vi "Begin.vi"(8 "error in":errorcluster) -> (0 "error out":errorcluster)   [LabVIEW 2017]
doc: "Called before other user functions, this VI is expected to open initial I/O refnums, load in file data, and do all program initialization. Notice that the <B>error out</B> terminal is simply used for data flow. Wiring it to other structures or subVIs ensures that this VI runs first."
uses:
  <vilib>/Rock Robotics/WPI/DriverStation/WPI_DriverStationRobotMode2.ctl
  <vilib>/Rock Robotics/WPI/Joystick/WPI_JoystickDeviceEnum.ctl
  <vilib>/Rock Robotics/WPI/ThirdParty/Phoenix-LabVIEW/Motor Controller/Controls/CTRE_Phoenix_MotorControl_ControlMode.ctl
  <vilib>/Rock Robotics/WPI/ThirdParty/Phoenix-LabVIEW/Motor Controller/Controls/CTRE_Phoenix_MotorControl_NeutralMode.ctl
  <vilib>/Rock Robotics/WPI/ThirdParty/Phoenix-LabVIEW/Motor Controller/Controls/CTRE_Phoenix_MotorControl_FeedbackDevice.ctl
  <vilib>/Rock Robotics/SystemInterfaces/spilib/spi_bus.ctl
  <vilib>/Rock Robotics/WPI/Solenoid/WPI_SolenoidChannel.ctl
  <vilib>/Rock Robotics/SystemInterfaces/DIO/FPGA_DIOChannel.ctl
  Robot Global Data.vi
  <vilib>/Rock Robotics/Network Tables/NT Write Numeric Array.vi
  <vilib>/Rock Robotics/WPI/Utilities/WPI_GetSetVariantRefNum.vi
  <vilib>/Rock Robotics/WPI/Gyro/WPI_GyroXRS450_SPI_Open.vi
  <vilib>/Rock Robotics/WPI/Switch/WPI_SwitchOpenLimit.vi
  <vilib>/Rock Robotics/WPI/Solenoid/WPI_SolenoidOpenDouble.vi
  <vilib>/Rock Robotics/Network Tables/NT Write String Array.vi
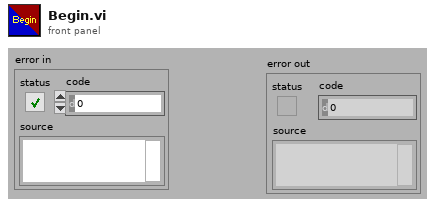
[diagram p1: front panel]
types:
  T1 = typedef "WPI_SolenoidChannel.ctl" = enum8{"Solenoid 0", "Solenoid 1", "Solenoid 2", "Solenoid 3", "Solenoid 4", "Solenoid 5", "Solenoid 6", "Solenoid 7", "Invalid"}
  T2 = typedef "FPGA_DIOChannel.ctl" = enum8{"DIO 0", "DIO 1", "DIO 2", "DIO 3", "DIO 4", "DIO 5", "DIO 6", "DIO 7", "DIO 8", "DIO 9", "DIO MXP 0", "DIO MXP 1", "DIO MXP 2", "DIO MXP 3", "DIO MXP 4", "DIO MXP 5", "DIO MXP 6", "DIO MXP 7", "DIO MXP 8", "DIO MXP 9", "DIO MXP 10", "DIO MXP 11", "DIO MXP 12", "DIO MXP 13", "DIO MXP 14", "DIO MXP 15", "SPI Port CS1", "SPI Port CS2", "SPI Port CS3", "SPI Port MISO", "SPI Port MOSI", "Invalid"}
  T3 = typedef "spi_bus.ctl" = enum16{"SPI On-Board, CS0", "SPI On-Board, CS1", "SPI On-Board, CS2", "SPI On-Board, CS3", "SPI MXP", "Invalid"}
  T4 = typedef "CTRE_Phoenix_MotorControl_FeedbackDevice.ctl" = i8
  T5 = typedef "CTRE_Phoenix_MotorControl_NeutralMode.ctl" = enum8{"EEPROMSetting", "Override to Coast", "Override to Brake"}
  T6 = typedef "CTRE_Phoenix_MotorControl_ControlMode.ctl" = u16
  T7 = typedef "WPI_JoystickDeviceEnum.ctl" = enum16{"USB 0", "USB 1", "USB 2", "USB 3", "USB 4", "USB 5"}
  T8 = typedef "WPI_DriverStationRobotMode2.ctl" = enum16{"Autonomous Disabled", "Autonomous Enabled", "Teleop Disabled", "Teleop Enabled", "Disconnected", "Finish", "Test Disabled", "Test Enabled", "Emergency Stopped"}
  T9 = typedef "WPI_SolenoidDevRef.ctl" = cluster{"DevStatus":errorcluster, "Pneumatics Control Module":u8, "Forward Solenoid Channel":T1, "Reverse Solenoid Channel":T1}
  T10 = typedef "WPI_JoystickDevRef.ctl" = cluster{"Device":T7}
  T11 = typedef "WPI_SwitchDevRef.ctl" = cluster{"DevStatus":errorcluster, "DIO Channel":T2, "CntIndex":T12, "Normally Closed":bool}
  T12 = typedef "FPGA_CounterCtrSystemIndex.ctl" = enum8{"Ctr 0", "Ctr 1", "Ctr 2", "Ctr 3", "Ctr 4", "Ctr 5", "Ctr 6", "Ctr 7", "Invalid"}
  T13 = typedef "WPI_MotorControlDeviceRef.ctl" = cluster{"DeviceStatus":errorcluster, "Type":T14, "PWM":cluster{"PWM Channel":T15, "DeadBand":T16}, "CAN":cluster{"Device Number":u8, "SetOutput VI Ref":variant, "GetOutput VI Ref":variant, "Enable VI Ref":variant, "Disable VI Ref":variant, "Data":variant}, "Invert":bool, "DIO PWM":cluster{"PWM \"Enable\" Channel":T15, "DIOChannel":T2, "PWM Rate":dbl}}
  T14 = typedef "WPI_MotorControlType.ctl" = enum16{"PWM", "CAN", "DIO PWM"}
  T15 = typedef "FPGA_DIOPWMChannel.ctl" = enum8{"PWM 0", "PWM 1", "PWM 2", "PWM 3", "PWM 4", "PWM 5", "PWM 6", "PWM 7", "PWM 8", "PWM 9", "PWM MXP 0", "PWM MXP 1", "PWM MXP 2", "PWM MXP 3", "PWM MXP 4", "PWM MXP 5", "PWM MXP 6", "PWM MXP 7", "PWM MXP 8", "PWM MXP 9", "Invalid"}
  T16 = typedef "WPI_PWMDeadband.ctl" = cluster{"Name":string, "maxPositivePwm":i32, "minPositivePwm":i32, "centerPwm":i32, "maxNegativePwm":i32, "minNegativePwm":i32, "angularRange":u16}
  T17 = typedef "WPI_GyroDevRef.ctl" = cluster{"DevStatus":errorcluster, "Analog Channel":T18, "Gain (VoltsPerDegree/Second)":dbl, "Gyro Type":enum16{"Analog", "XRS450"}, "Handle":i32, "SPI Bus":T3, "Device Found":bool, "Sample Rate":dbl, "Calibrate On Open":bool, "Offset":dbl}
  T18 = typedef "FPGA_AIChannel.ctl" = enum8{"AI 0", "AI 1", "AI 2", "AI 3", "AI MXP 0", "AI MXP 1", "AI MXP 2", "AI MXP 3", "Invalid"}
  T19 = typedef "WPI_CompressorDevRef.ctl" = cluster{"DevStatus":errorcluster, "Pneumatics Control Module":u8}
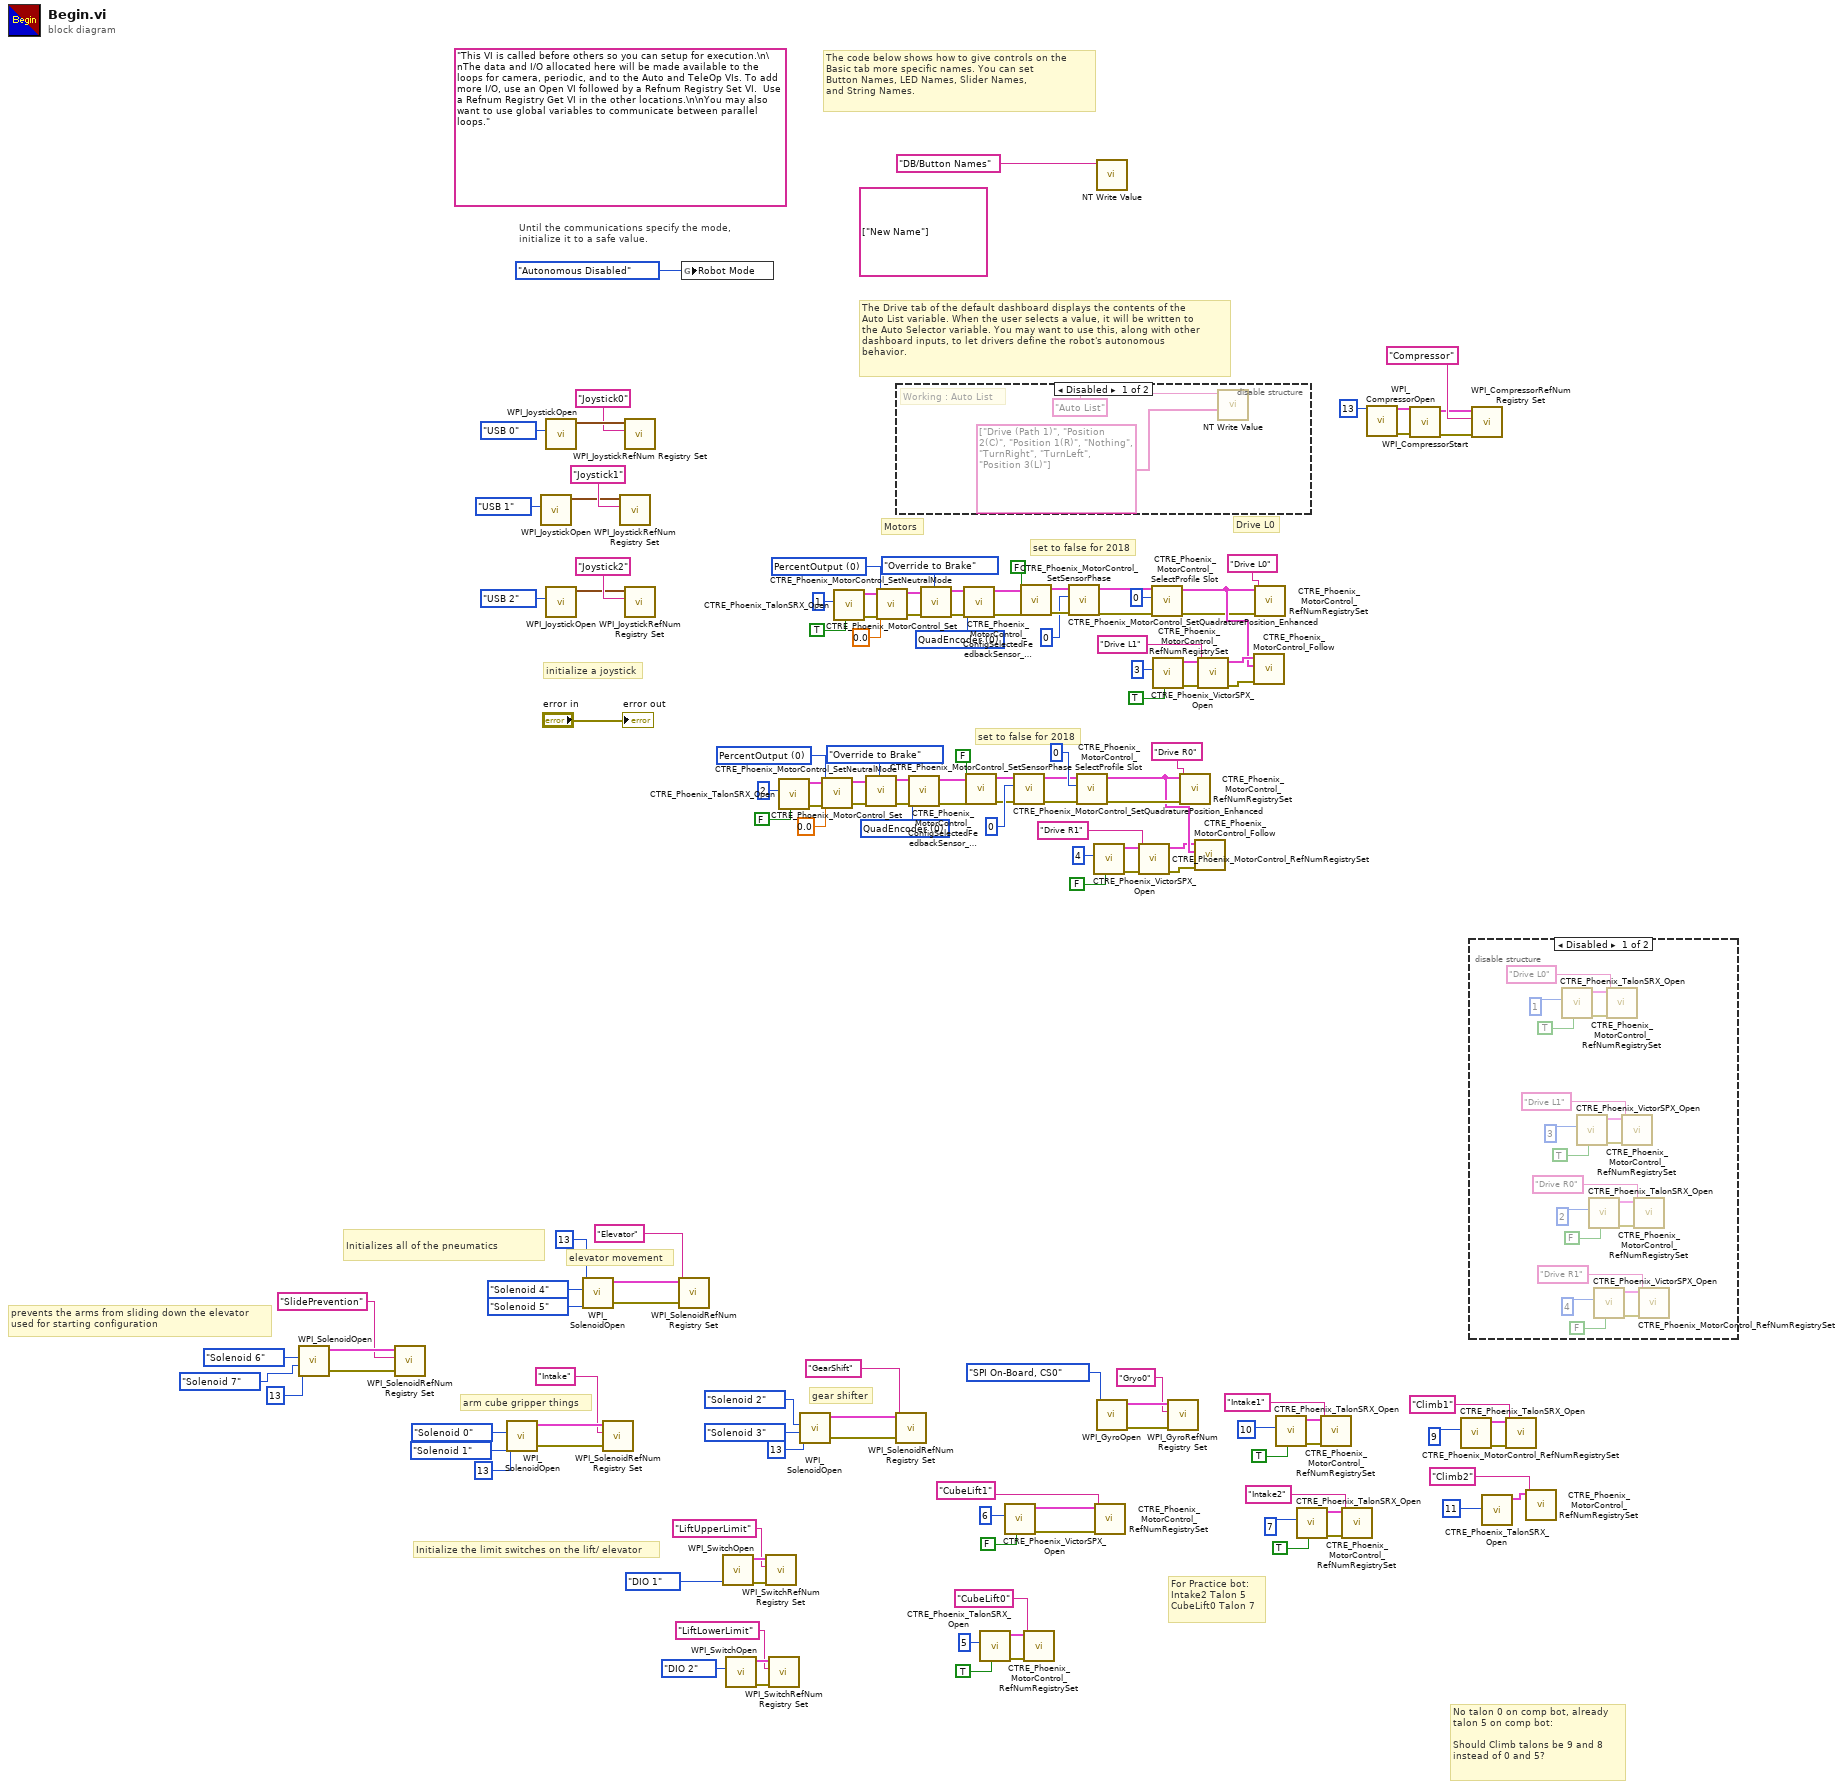
[diagram p0: block diagram]
diagram:
  w93 = T4 0 items=["None"=-1, "QuadEncoder"=0, "Analog"=2, "Tachometer"=4, "Pulse Width Encoded Position"=8, "Sensor Sum (S0 + S1)"=9, "Sensor Difference (D0 - D1)"=10, "Remote Source 0"=11, "Remote Source 1"=12, "Software Emulated"=15] ("Feedback Device")
  w88 = T6 0 items=["PercentOutput"=0, "Position"=1, "Velocity"=2, "Current"=3, "Follower"=5, "MotionProfile"=6, "MotionMagic"=7, "MotionMagicArc"=8, "MotionProfileArc"=10, "Disabled"=15] ("Control Mode")
  w112 = T4 0 items=["None"=-1, "QuadEncoder"=0, "Analog"=2, "Tachometer"=4, "Pulse Width Encoded Position"=8, "Sensor Sum (S0 + S1)"=9, "Sensor Difference (D0 - D1)"=10, "Remote Source 0"=11, "Remote Source 1"=12, "Software Emulated"=15] ("Feedback Device")
  w117 = T6 0 items=["PercentOutput"=0, "Position"=1, "Velocity"=2, "Current"=3, "Follower"=5, "MotionProfile"=6, "MotionMagic"=7, "MotionMagicArc"=8, "MotionProfileArc"=10, "Disabled"=15] ("Control Mode")
  (unwired) string[] ["New Name"]
  (unwired) "This VI is called before others so you can setup for execution.\n\nThe data and I/O allocated here will be made available to the loops for camera, periodic, and to the Auto and TeleOp VIs. To add more I/O, use an Open VI followed by a Refnum Registry Set VI.  Use a Refnum Registry Get VI in the other locations.\n\nYou may also want to use global variables to communicate between parallel loops."
  # "prevents the arms from sliding down the elevator\nused for starting configuration"
  # "No talon 0 on comp bot, already\ntalon 5 on comp bot:\n\nShould Climb talons be 9 and 8\ninstead of 0 and 5?"
  # "gear shifter"
  # "arm cube gripper things"
  # "elevator movement"
  # "Initialize the limit switches on the lift/ elevator"
  # "Initializes all of the pneumatics"
  # "For Practice bot:\nIntake2 Talon 5\nCubeLift0 Talon 7"
  # "set to false for 2018"
  # "set to false for 2018"
  # "Drive L0"
  # "Motors"
  # "The Drive tab of the default dashboard displays the contents of the\nAuto List variable. When the user selects a value, it will be written to\nthe Auto Selector variable. You may want to use this, along with other\ndashboard inputs, to let drivers define the robot's autonomous\nbehavior."
  # "The code below shows how to give controls on the\nBasic tab more specific names. You can set\nButton Names, LED Names, Slider Names,\nand String Names."
  # "initialize a joystick"
  # "Until the communications specify the mode,\ninitialize it to a safe value."
  n1 = call-poly <vilib>:"WPI_SolenoidOpen.vi"("Reverse Solenoid Channel"=WPI_SolenoidChannel."Solenoid 7" ("Forward Solenoid Channel"), "Forward Solenoid Channel"=WPI_SolenoidChannel."Solenoid 6", "Pneumatics Control Module (0)"=u8 13) -> ("error out"=w5:errorcluster, "SolenoidDevRef"=w7:T9)  [unwired: 7 in]
  n2 = call <vilib>:"WPI_SolenoidRefNum Registry Set.vi"("error in (no error)"=w5, "refnum name"="SlidePrevention", "SolenoidDevRef"=w7) -> ()  [unwired: 7 in, 2 out]
  n3 = call-poly <vilib>:"WPI_SolenoidOpen.vi"("Reverse Solenoid Channel"=WPI_SolenoidChannel."Solenoid 1", "Forward Solenoid Channel"=WPI_SolenoidChannel."Solenoid 0", "Pneumatics Control Module (0)"=u8 13) -> ("error out"=w8:errorcluster, "SolenoidDevRef"=w30:T9)  [unwired: 7 in]
  n4 = call <vilib>:"WPI_JoystickOpen.vi"("JoystickDevice"=WPI_JoystickDeviceEnum."USB 1") -> ("JoystickDevRef"=w141:T10)  [unwired: 10 in]
  n5 = call <vilib>:"WPI_JoystickOpen.vi"("JoystickDevice"=WPI_JoystickDeviceEnum."USB 0") -> ("JoystickDevRef"=w136:T10)  [unwired: 10 in]
  n6 = call <vilib>:"WPI_JoystickOpen.vi"("JoystickDevice"=WPI_JoystickDeviceEnum."USB 2") -> ("JoystickDevRef"=w133:T10)  [unwired: 10 in]
  n7 = call-poly <vilib>:"WPI_SolenoidOpen.vi"("Reverse Solenoid Channel"=WPI_SolenoidChannel."Solenoid 5", "Forward Solenoid Channel"=WPI_SolenoidChannel."Solenoid 4", "Pneumatics Control Module (0)"=u8 13) -> ("error out"=w38:errorcluster, "SolenoidDevRef"=w37:T9)  [unwired: 7 in]
  n8 = call <vilib>:"WPI_SolenoidRefNum Registry Set.vi"("error in (no error)"=w8, "refnum name"="Intake", "SolenoidDevRef"=w30) -> ()  [unwired: 7 in, 2 out]
  n9 = call <vilib>:"WPI_JoystickRefNum Registry Set.vi"("refnum name"="Joystick1", "JoystickDevRef"=w141) -> ()  [unwired: 8 in, 2 out]
  n10 = call <vilib>:"WPI_JoystickRefNum Registry Set.vi"("refnum name"="Joystick0", "JoystickDevRef"=w136) -> ()  [unwired: 8 in, 2 out]
  n11 = call <vilib>:"WPI_JoystickRefNum Registry Set.vi"("refnum name"="Joystick2", "JoystickDevRef"=w133) -> ()  [unwired: 8 in, 2 out]
  n12 = call <vilib>:"WPI_SolenoidRefNum Registry Set.vi"("error in (no error)"=w38, "refnum name"="Elevator", "SolenoidDevRef"=w37) -> ()  [unwired: 7 in, 2 out]
  n13 = global write "Robot Global Data.vi" "Robot Mode"(WPI_DriverStationRobotMode2."Autonomous Disabled" ("Robot Mode")) -> ()
  n14 = call-poly <vilib>:"WPI_SwitchOpen.vi"("DIO Channel"=FPGA_DIOChannel."DIO 1") -> ("error out"=w27:errorcluster, "SwitchDevRef"=w26:T11)  [unwired: 9 in]
  n15 = call-poly <vilib>:"WPI_SwitchOpen.vi"("DIO Channel"=FPGA_DIOChannel."DIO 2") -> ("error out"=w24:errorcluster, "SwitchDevRef"=w23:T11)  [unwired: 9 in]
  n16 = call <vilib>:"WPI_SwitchRefNum Registry Set.vi"("error in (no error)"=w27, "refnum name"="LiftUpperLimit", "SwitchDevRef"=w26) -> ()  [unwired: 7 in, 2 out]
  n17 = call <vilib>:"WPI_SwitchRefNum Registry Set.vi"("error in (no error)"=w24, "refnum name"="LiftLowerLimit", "SwitchDevRef"=w23) -> ()  [unwired: 7 in, 2 out]
  n18 = call "CTRE_Phoenix_TalonSRX_Open.vi"("Invert"=FALSE, "Device Number"=u8 2) -> ("error out"=w85:errorcluster, "CAN Talon SRX Ref"=w84:T13)  [unwired: 8 in]
  n19 = call-poly <vilib>:"WPI_SolenoidOpen.vi"("Reverse Solenoid Channel"=WPI_SolenoidChannel."Solenoid 3", "Forward Solenoid Channel"=WPI_SolenoidChannel."Solenoid 2", "Pneumatics Control Module (0)"=u8 13) -> ("error out"=w31:errorcluster, "SolenoidDevRef"=w32:T9)  [unwired: 7 in]
  n20 = call <vilib>:"CTRE_Phoenix_MotorControl_Set.vi"("error in (no error)"=w85, "Output"=0.0, "Control Mode"=w88, "PhoenixMotorControlDevRef"=w84) -> ("error out"=w87:errorcluster, "PhoenixMotorControlDevRef"=w86:T13)  [unwired: 6 in]
  n21 = call "CTRE_Phoenix_TalonSRX_Open.vi"("Invert"=TRUE, "Device Number"=u8 1) -> ("error out"=w120:errorcluster, "CAN Talon SRX Ref"=w121:T13)  [unwired: 8 in]
  n22 = call <vilib>:"CTRE_Phoenix_MotorControl_SetNeutralMode.vi"("error in (no error)"=w87, "Motor Control Neutral Mode"=CTRE_Phoenix_MotorControl_NeutralMode."Override to Brake", "PhoenixMotorControlDevRef"=w86) -> ("error out"=w91:errorcluster, "PhoenixMotorControlDevRef"=w92:T13)  [unwired: 7 in]
  n23 = call <vilib>:"CTRE_Phoenix_MotorControl_Set.vi"("error in (no error)"=w120, "Output"=0.0, "Control Mode"=w117, "PhoenixMotorControlDevRef"=w121) -> ("error out"=w118:errorcluster, "PhoenixMotorControlDevRef"=w119:T13)  [unwired: 6 in]
  n24 = call <vilib>:"WPI_SolenoidRefNum Registry Set.vi"("error in (no error)"=w31, "refnum name"="GearShift", "SolenoidDevRef"=w32) -> ()  [unwired: 7 in, 2 out]
  n25 = disable-structure shown="Disabled" {
    frame Disabled {
      # "Working : Auto List"
      n26 = call-poly <vilib>:"NT Write Value.vi"("String Array"=string[] ["Drive (Path 1)", "Position 2(C)", "Position 1(R)", "Nothing", "TurnRight", "TurnLeft", "Position 3(L)"], "Name"="Auto List") -> ()  [unwired: 9 in, 1 out]
    }
    frame Enabled {
    }
  }
  n27 = call <vilib>:"CTRE_Phoenix_MotorControl_ConfigSelectedFeedbackSensor_Enhanced.vi"("error in (no error)"=w91, "Feedback Device"=w93, "PhoenixMotorControlDevRef"=w92) -> ("error out"=w95:errorcluster, "PhoenixMotorControlDevRef"=w94:T13)  [unwired: 7 in]
  n28 = call <vilib>:"CTRE_Phoenix_MotorControl_SetNeutralMode.vi"("error in (no error)"=w118, "Motor Control Neutral Mode"=CTRE_Phoenix_MotorControl_NeutralMode."Override to Brake", "PhoenixMotorControlDevRef"=w119) -> ("error out"=w114:errorcluster, "PhoenixMotorControlDevRef"=w113:T13)  [unwired: 7 in]
  n29 = call <vilib>:"CTRE_Phoenix_MotorControl_ConfigSelectedFeedbackSensor_Enhanced.vi"("error in (no error)"=w114, "Feedback Device"=w112, "PhoenixMotorControlDevRef"=w113) -> ("error out"=w110:errorcluster, "PhoenixMotorControlDevRef"=w111:T13)  [unwired: 7 in]
  n30 = call <vilib>:"CTRE_Phoenix_MotorControl_SetSensorPhase.vi"("error in (no error)"=w95, "PhaseSensor"=FALSE, "PhoenixMotorControlDevRef"=w94) -> ("error out"=w97:errorcluster, "PhoenixMotorControlDevRef"=w98:T13)  [unwired: 7 in]
  n31 = call "CTRE_Phoenix_TalonSRX_Open.vi"("Invert"=TRUE, "Device Number"=u8 5) -> ("error out"=w50:errorcluster, "CAN Talon SRX Ref"=w49:T13)  [unwired: 8 in]
  n32 = call <vilib>:"CTRE_Phoenix_VictorSPX_Open.vi"("Invert"=FALSE, "Device Number"=u8 6) -> ("error out"=w53:errorcluster, "CAN Talon SRX Ref"=w52:T13)  [unwired: 8 in]
  n33 = call <vilib>:"CTRE_Phoenix_MotorControl_SetQuadraturePosition_Enhanced.vi"("error in (no error)"=w97, "New Position"=0, "PhoenixMotorControlDevRef"=w98) -> ("error out"=w11:errorcluster, "PhoenixMotorControlDevRef"=w12:T13)  [unwired: 7 in]
  n34 = call <vilib>:"CTRE_Phoenix_MotorControl_SetSensorPhase.vi"("error in (no error)"=w110, "PhaseSensor"=FALSE, "PhoenixMotorControlDevRef"=w111) -> ("error out"=w108:errorcluster, "PhoenixMotorControlDevRef"=w107:T13)  [unwired: 7 in]
  n35 = call <vilib>:"CTRE_Phoenix_MotorControl_RefNumRegistrySet.vi"("error in (no error)"=w50, "refnum name"="CubeLift0", "PhoenixMotorControlDevRef"=w49) -> ()  [unwired: 7 in, 2 out]
  n36 = call <vilib>:"CTRE_Phoenix_MotorControl_SetQuadraturePosition_Enhanced.vi"("error in (no error)"=w108, "New Position"=0, "PhoenixMotorControlDevRef"=w107) -> ("error out"=w13:errorcluster, "PhoenixMotorControlDevRef"=w14:T13)  [unwired: 7 in]
  n37 = call <vilib>:"CTRE_Phoenix_MotorControl_SelectProfile Slot.vi"("error in (no error)"=w11, "slotIdx"=0, "PhoenixMotorControlDevRef"=w12) -> ("error out"=w101:errorcluster, "PhoenixMotorControlDevRef"=w100:T13)  [unwired: 7 in]
  n38 = call <vilib>:"CTRE_Phoenix_VictorSPX_Open.vi"("Invert"=FALSE, "Device Number"=u8 4) -> ("error out"=w77:errorcluster, "CAN Talon SRX Ref"=w78:T13)  [unwired: 8 in]
  n39 = call <vilib>:"CTRE_Phoenix_MotorControl_RefNumRegistrySet.vi"("error in (no error)"=w53, "refnum name"="CubeLift1", "PhoenixMotorControlDevRef"=w52) -> ()  [unwired: 7 in, 2 out]
  n40 = call-poly <vilib>:"NT Write Value.vi"("Name"="DB/Button Names") -> ()  [unwired: 10 in, 1 out]
  n41 = call-poly <vilib>:"WPI_GyroOpen.vi"("SPI Bus"=spi_bus."SPI On-Board, CS0") -> ("error out"=w45:errorcluster, "GyroDevRef"=w46:T17)  [unwired: 8 in, 1 out]
  n42 = call <vilib>:"CTRE_Phoenix_MotorControl_RefNumRegistrySet.vi"("error in (no error)"=w77, "refnum name"="Drive R1", "PhoenixMotorControlDevRef"=w78) -> ("error out"=w80:errorcluster, "PhoenixMotorControlDevRef"=w81:T13)  [unwired: 7 in]
  n43 = call <vilib>:"CTRE_Phoenix_MotorControl_SelectProfile Slot.vi"("error in (no error)"=w13, "slotIdx"=0, "PhoenixMotorControlDevRef"=w14) -> ("error out"=w104:errorcluster, "PhoenixMotorControlDevRef"=w105:T13)  [unwired: 7 in]
  n44 = call <vilib>:"CTRE_Phoenix_VictorSPX_Open.vi"("Invert"=TRUE, "Device Number"=u8 3) -> ("error out"=w128:errorcluster, "CAN Talon SRX Ref"=w127:T13)  [unwired: 8 in]
  n45 = call <vilib>:"WPI_GyroRefNum Registry Set.vi"("error in (no error)"=w45, "refnum name"="Gryo0", "GyroDevRef"=w46) -> ()  [unwired: 7 in, 2 out]
  n46 = call <vilib>:"CTRE_Phoenix_MotorControl_RefNumRegistrySet.vi"("error in (no error)"=w101, "refnum name"="Drive R0", "PhoenixMotorControlDevRef"=w100) -> ()  [unwired: 7 in, 2 out]
  n47 = call <vilib>:"CTRE_Phoenix_MotorControl_Follow.vi"("error in (no error)"=w80, "Master Controller to Follow"=w100, "PhoenixMotorControlDevRef"=w81) -> ()  [unwired: 7 in, 2 out]
  n48 = call <vilib>:"CTRE_Phoenix_MotorControl_RefNumRegistrySet.vi"("error in (no error)"=w128, "refnum name"="Drive L1", "PhoenixMotorControlDevRef"=w127) -> ("error out"=w125:errorcluster, "PhoenixMotorControlDevRef"=w124:T13)  [unwired: 7 in]
  n49 = call <vilib>:"CTRE_Phoenix_MotorControl_Follow.vi"("error in (no error)"=w125, "Master Controller to Follow"=w105, "PhoenixMotorControlDevRef"=w124) -> ()  [unwired: 7 in, 2 out]
  n50 = call <vilib>:"CTRE_Phoenix_MotorControl_RefNumRegistrySet.vi"("error in (no error)"=w104, "refnum name"="Drive L0", "PhoenixMotorControlDevRef"=w105) -> ()  [unwired: 7 in, 2 out]
  n51 = call "CTRE_Phoenix_TalonSRX_Open.vi"("Invert"=TRUE, "Device Number"=u8 10) -> ("error out"=w62:errorcluster, "CAN Talon SRX Ref"=w61:T13)  [unwired: 8 in]
  n52 = call "CTRE_Phoenix_TalonSRX_Open.vi"("Invert"=TRUE, "Device Number"=u8 7) -> ("error out"=w58:errorcluster, "CAN Talon SRX Ref"=w57:T13)  [unwired: 8 in]
  n53 = call <vilib>:"CTRE_Phoenix_MotorControl_RefNumRegistrySet.vi"("error in (no error)"=w62, "refnum name"="Intake1", "PhoenixMotorControlDevRef"=w61) -> ()  [unwired: 7 in, 2 out]
  n54 = call <vilib>:"CTRE_Phoenix_MotorControl_RefNumRegistrySet.vi"("error in (no error)"=w58, "refnum name"="Intake2", "PhoenixMotorControlDevRef"=w57) -> ()  [unwired: 7 in, 2 out]
  n55 = call <vilib>:"WPI_CompressorOpen.vi"("Pneumatics Control Module (0)"=u8 13) -> ("CompressorDevRef"=w72:T19, "error out"=w71:errorcluster)  [unwired: 13 in]
  n56 = call <vilib>:"WPI_CompressorStart.vi"("error in (no error)"=w71, "CompressorDevRef"=w72) -> ("error out"=w69:errorcluster, "CompressorDevRef"=w70:T19)  [unwired: 8 in]
  n57 = call "CTRE_Phoenix_TalonSRX_Open.vi"("Device Number"=u8 9) -> ("error out"=w67:errorcluster, "CAN Talon SRX Ref"=w66:T13)  [unwired: 9 in]
  n58 = disable-structure shown="Disabled" {
    frame Disabled {
      n59 = call "CTRE_Phoenix_TalonSRX_Open.vi"("Invert"=TRUE, "Device Number"=u8 1) -> ("error out"=w162:errorcluster, "CAN Talon SRX Ref"=w163:T13)  [unwired: 8 in]
      n60 = call <vilib>:"CTRE_Phoenix_VictorSPX_Open.vi"("Invert"=TRUE, "Device Number"=u8 3) -> ("error out"=w161:errorcluster, "CAN Talon SRX Ref"=w160:T13)  [unwired: 8 in]
      n61 = call "CTRE_Phoenix_TalonSRX_Open.vi"("Invert"=FALSE, "Device Number"=u8 2) -> ("error out"=w154:errorcluster, "CAN Talon SRX Ref"=w155:T13)  [unwired: 8 in]
      n62 = call <vilib>:"CTRE_Phoenix_VictorSPX_Open.vi"("Invert"=FALSE, "Device Number"=u8 4) -> ("error out"=w153:errorcluster, "CAN Talon SRX Ref"=w152:T13)  [unwired: 8 in]
      n63 = call <vilib>:"CTRE_Phoenix_MotorControl_RefNumRegistrySet.vi"("error in (no error)"=w162, "refnum name"="Drive L0", "PhoenixMotorControlDevRef"=w163) -> ()  [unwired: 7 in, 2 out]
      n64 = call <vilib>:"CTRE_Phoenix_MotorControl_RefNumRegistrySet.vi"("error in (no error)"=w161, "refnum name"="Drive L1", "PhoenixMotorControlDevRef"=w160) -> ()  [unwired: 7 in, 2 out]
      n65 = call <vilib>:"CTRE_Phoenix_MotorControl_RefNumRegistrySet.vi"("error in (no error)"=w154, "refnum name"="Drive R0", "PhoenixMotorControlDevRef"=w155) -> ()  [unwired: 7 in, 2 out]
      n66 = call <vilib>:"CTRE_Phoenix_MotorControl_RefNumRegistrySet.vi"("error in (no error)"=w153, "refnum name"="Drive R1", "PhoenixMotorControlDevRef"=w152) -> ()  [unwired: 7 in, 2 out]
    }
    frame Enabled {
    }
  }
  n67 = call <vilib>:"WPI_CompressorRefNum Registry Set.vi"("error in (no error)"=w69, "refnum name"="Compressor", "CompressorDevRef"=w70) -> ()  [unwired: 7 in, 2 out]
  n68 = call "CTRE_Phoenix_TalonSRX_Open.vi"("Device Number"=u8 11) -> ("CAN Talon SRX Ref"=w9:T13)  [unwired: 9 in, 1 out]
  n69 = call <vilib>:"CTRE_Phoenix_MotorControl_RefNumRegistrySet.vi"("error in (no error)"=w67, "refnum name"="Climb1", "PhoenixMotorControlDevRef"=w66) -> ()  [unwired: 7 in, 2 out]
  n70 = call <vilib>:"CTRE_Phoenix_MotorControl_RefNumRegistrySet.vi"("refnum name"="Climb2", "PhoenixMotorControlDevRef"=w9) -> ()  [unwired: 8 in, 2 out]
  "error out" <- "error in"
